vi "Write FPGA Interface.vi"(8 "error in (no error)":errorcluster, 10 "FPGA Interface":refnum<k20>, 11 "FPGA-Bus in":refnum<class "FPGA-Bus.lvclass">) -> (0 "error out":errorcluster, 3 "FPGA-Bus out":refnum<class "FPGA-Bus.lvclass">)   [LabVIEW 2021, in "FPGA-Bus.lvclass"]
uses:
  FPGA-Bus.lvclass
  FPGA-Bus.lvclass/FPGA-Bus.ctl
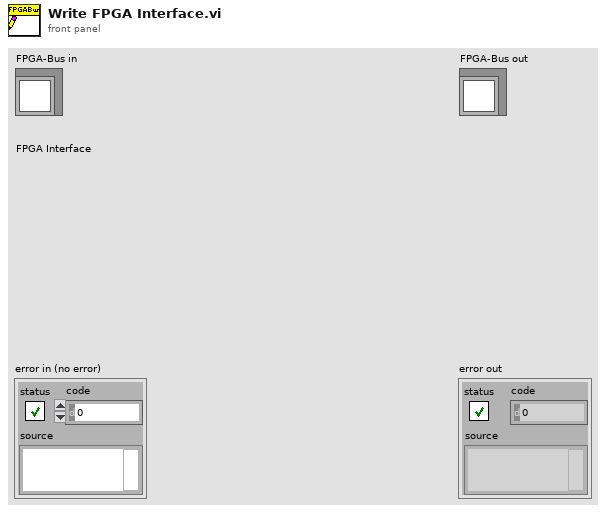
[diagram p1: front panel]
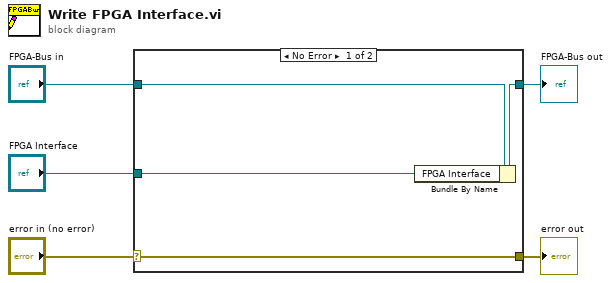
[diagram p0: block diagram]
diagram:
  n1 = case shown="No Error" "error in (no error)" {
    selector: "error in (no error)" -> [w9 w10]
    tunnel: [w9 w10] -> w4
    tunnel: [w7 w11] -> w2
    tunnel: "FPGA-Bus in" -> [w8 w11]
    tunnel: "FPGA Interface" -> [w6 _]
    frame No Error {
      n2 = Bundle By Name(cluster=w8, "FPGA Interface"=w6) -> (w7:refnum<class "FPGA-Bus.lvclass">)
    }
    frame Error {
    }
  }
  "error out" <- w4
  "FPGA-Bus out" <- w2
